vi "DHE_GetProgress.vi"(10 "phys. unit":string, 11 "Databse Ref":T1) -> (2 "progress":string)   [LabVIEW 2016]
uses:
  DBSHAND/private/vis/DatabaseHand_RefNum.ctl
  Common/public/vis/CMN_FVAR_action.ctl
  DBSHAND/private/vis/DatabaseHand_Element_Get(string).vi
  DBSHAND/private/vis/DatabaseHand_Element_Get(U8).vi
  DBSHAND/private/vis/DatabaseHand_Element_Get(double).vi
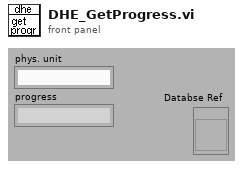
[diagram p1: front panel]
types:
  T1 = typedef "DatabaseHand_RefNum.ctl" = refnum<vi>
  T2 = typedef "CMN_FVAR_action.ctl" = enum16{"read", "write"}
  T3 = enum16{"Idle", "Exposing", "Paused", "AbortExp", "Reading", "AbortRead", "FinishedReading", "Resetting", "Reducing", "Initializing"}
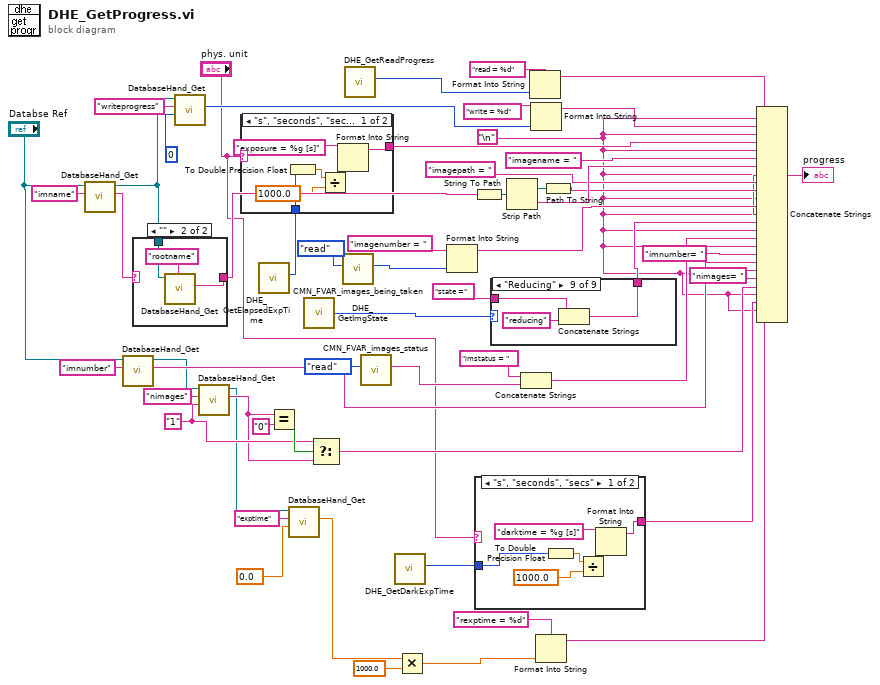
[diagram p0: block diagram]
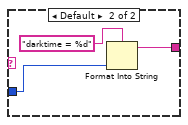
[diagram p2: hidden frame]
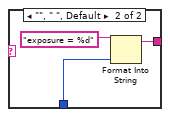
[diagram p4: hidden frame]
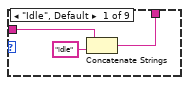
[diagram p5: hidden frame]
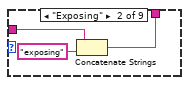
[diagram p6: hidden frame]
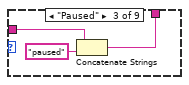
[diagram p7: hidden frame]
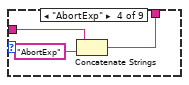
[diagram p8: hidden frame]
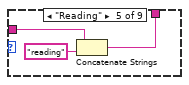
[diagram p9: hidden frame]
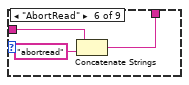
[diagram p10: hidden frame]
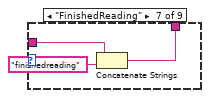
[diagram p11: hidden frame]
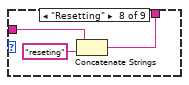
[diagram p12: hidden frame]
diagram:
  w26 = "1"
  w1 = "\n"
  n1 = call-poly "DatabaseHand_Get.vi"("name"="imname", "Database RefNum in"="Databse Ref") -> ("value"=w22:string, "Database RefNum out"=w20:T1)  [unwired: 3 in, 5 out]
  n2 = call-poly "DatabaseHand_Get.vi"("name"="imnumber", "Database RefNum in"="Databse Ref") -> ("value"=w31:string, "Database RefNum out"=w30:T1)  [unwired: 3 in, 5 out]
  n3 = case shown="\"\"" w22 {
    selector: w22 -> [w57 _]
    tunnel: [w57 w58] -> w21
    tunnel: w20 -> [_ w60]
    frame Default {
    }
    frame "" {
      n4 = call-poly "DatabaseHand_Get.vi"("name"="rootname", "Database RefNum in"=w60) -> ("value"=w58:string)  [unwired: 3 in, 6 out]
    }
  }
  n5 = call-poly "DatabaseHand_Get.vi"("default value"=u8 0 ("Writeprogress"), "name"="writeprogress", "Database RefNum in"=w20) -> ("value"=w35:u8)  [unwired: 2 in, 6 out]
  n6 = call-poly "DatabaseHand_Get.vi"("default value"=w26, "name"="nimages", "Database RefNum in"=w30) -> ("value"=w25:string, "Database RefNum out"=w9:T1)  [unwired: 2 in, 5 out]
  n7 = call "DHE_GetElapsedExpTime.vi"() -> ("ElapsedExp"=w18:u32)  [unwired: 11 out]
  n8 = case shown="\"s\", \"seconds\", \"secs\"" "phys. unit" {
    tunnel: [w65 w68] -> w51
    tunnel: w18 -> [w64 w67]
    frame "s", "seconds", "secs" {
      n9 = To Double Precision Float(number=w64) -> (double precision float=w63:dbl)
      n10 = Divide(x=w63, y=1000.0) -> (x/y=w61:dbl)
      n11 = Format Into String(format string="exposure = %g [s]", w61) -> (resulting string=w65:string)  [unwired: 2 in, 1 out]
    }
    frame "", " ", Default {
      n12 = Format Into String(format string="exposure = %d", w67) -> (resulting string=w68:string)  [unwired: 2 in, 1 out]
    }
  }
  n13 = Equal?(x=w25, y="0") -> (x = y?=w27:bool)
  n14 = call-poly "DatabaseHand_Get.vi"("default value"=0.0 ("y"), "name"="exptime", "Database RefNum in"=w9) -> ("value"=w6:dbl)  [unwired: 2 in, 6 out]
  n15 = call "DHE_GetImgState.vi"() -> ("DHE_ImgState"=w19:T3)  [unwired: 9 out]
  n16 = Select(t=w26, s=w27, f=w25) -> (s? t:f=w23:string)
  n17 = call "CMN_FVAR_images_being_taken.vi"("action"=CMN_FVAR_action."read") -> ("value out"=w16:i32)  [unwired: 1 in, 8 out]
  n18 = call "DHE_GetReadProgress.vi"() -> ("ReadProgress"=w17:u32)  [unwired: 11 out]
  n19 = call "CMN_FVAR_images_status.vi"("action"=CMN_FVAR_action."read") -> ("value out"=w14:string)  [unwired: 1 in, 8 out]
  n20 = call "DHE_GetDarkExpTime.vi"() -> ("DarkExp"=w11:u32)  [unwired: 11 out]
  n21 = Multiply(x=w6, y=1000.0) -> (x*y=w4:dbl)
  n22 = Format Into String(initial string="imagenumber = " ("string"), w16) -> (resulting string=w42:string)  [unwired: 2 in, 1 out]
  n23 = String To Path(string=w21) -> (path=w49:path)
  n24 = case shown="\"s\", \"seconds\", \"secs\"" "phys. unit" {
    tunnel: w11 -> [w71 w78]
    tunnel: [w70 w76] -> w10
    frame "s", "seconds", "secs" {
      n25 = To Double Precision Float(number=w71) -> (double precision float=w74:dbl)
      n26 = Divide(x=w74, y=1000.0) -> (x/y=w72:dbl)
      n27 = Format Into String(format string="darktime = %g [s]", w72) -> (resulting string=w70:string)  [unwired: 2 in, 1 out]
    }
    frame Default {
      n28 = Format Into String(format string="darktime = %d", w78) -> (resulting string=w76:string)  [unwired: 2 in, 1 out]
    }
  }
  n29 = case shown="\"Reducing\"" w19 {
    tunnel: "state =" -> [w80 w84 w87 w90 w93 w96 w99 w102 w105]
    tunnel: [w79 w82 w85 w88 w91 w94 w97 w100 w103] -> w44
    frame "Idle", Default {
      n30 = Concatenate Strings(w80, "idle" ("string")) -> (w79:string)
    }
    frame "Exposing" {
      n31 = Concatenate Strings(w84, "exposing" ("string")) -> (w82:string)
    }
    frame "Paused" {
      n32 = Concatenate Strings(w87, "paused" ("string")) -> (w85:string)
    }
    frame "AbortExp" {
      n33 = Concatenate Strings(w90, "AbortExp" ("string")) -> (w88:string)
    }
    frame "Reading" {
      n34 = Concatenate Strings(w93, "reading" ("string")) -> (w91:string)
    }
    frame "AbortRead" {
      n35 = Concatenate Strings(w96, "abortread" ("string")) -> (w94:string)
    }
    frame "FinishedReading" {
      n36 = Concatenate Strings(w99, "finishedreading" ("string")) -> (w97:string)
    }
    frame "Resetting" {
      n37 = Concatenate Strings(w102, "reseting" ("string")) -> (w100:string)
    }
    frame "Reducing" {
      n38 = Concatenate Strings(w105, "reducing" ("string")) -> (w103:string)
    }
  }
  n39 = Strip Path(path=w49) -> (stripped path=w47:path, name=w48:string)
  n40 = Concatenate Strings("imstatus = " ("string"), w14) -> (w40:string)
  n41 = Format Into String(format string="read = %d", w17) -> (resulting string=w54:string)  [unwired: 2 in, 1 out]
  n42 = Format Into String(format string="write = %d", w35) -> (resulting string=w52:string)  [unwired: 2 in, 1 out]
  n43 = Format Into String(format string="rexptime = %d", w4) -> (resulting string=w2:string)  [unwired: 2 in, 1 out]
  n44 = Path To String(path=w47) -> (string=w45:string)
  n45 = Concatenate Strings(w54, w1, w52, w1, w51, w1, "imagename = " ("string"), w48, w1, "imagepath = " ("string"), w45, w1, w42, w1, w44, w1, w40, w1, "imnumber= " ("string"), w31, w1, "nimages= " ("string"), w23, w1, w10, w1, w2) -> (→"progress":string)
